vi "Write ADU Packet.vi"(8 "error in":errorcluster, 9 "modbus data unit":refnum<class "Modbus Data Unit.lvclass">, 10 "isMaster (f)":bool, 11 "ASCII transmission data unit in":refnum<class "ASCII Data Unit.lvclass">) -> (0 "error out":errorcluster, 3 "ASCII transmission data unit out":refnum<class "ASCII Data Unit.lvclass">)   [LabVIEW 2021, in "ASCII Data Unit.lvclass"]
uses:
  ASCII Data Unit.lvclass
  D:/my_projects/projects/Algorithms/Labview/21/Modbus_v121c/Transmission Data Unit/Serial Interface/Serial Data Unit.lvclass
  D:/my_projects/projects/Algorithms/Labview/21/Modbus_v121c/Transmission Data Unit/Transmission Data Unit.lvclass
  Modbus Data Unit/Modbus Data Unit.lvclass
  Modbus Data Unit/Modbus Data Unit.lvclass/Modbus Data Unit.ctl
  Serial Interface/Serial Data Unit.lvclass/Serial Data Unit.ctl
  Transmission Data Unit.lvclass/Transmission Data Unit.ctl
  <vilib>/Utility/error.llb/Error Cluster From Error Code.vi
  <vilib>/ErrorRing/Error Ring.xnode
  ASCII Data Unit.lvclass/ASCII Data Unit.ctl
  Serial Interface/Serial Data Unit.lvclass
  Transmission Data Unit.lvclass
  Network Interface/Serial Interface/Serial Shared Components/Serial Shared Components.lvlib
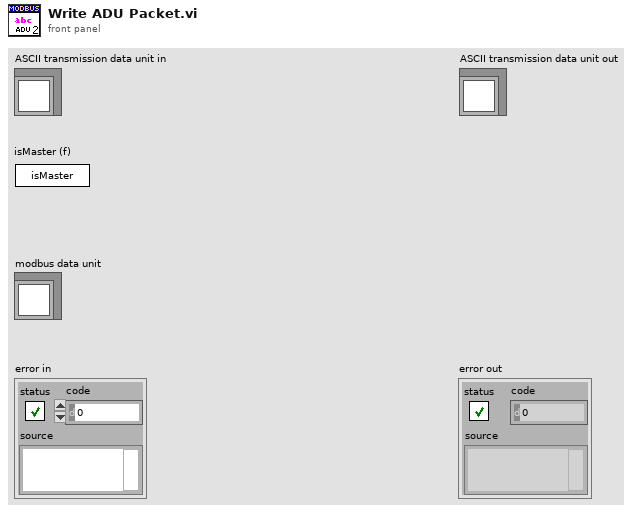
[diagram p1: front panel]
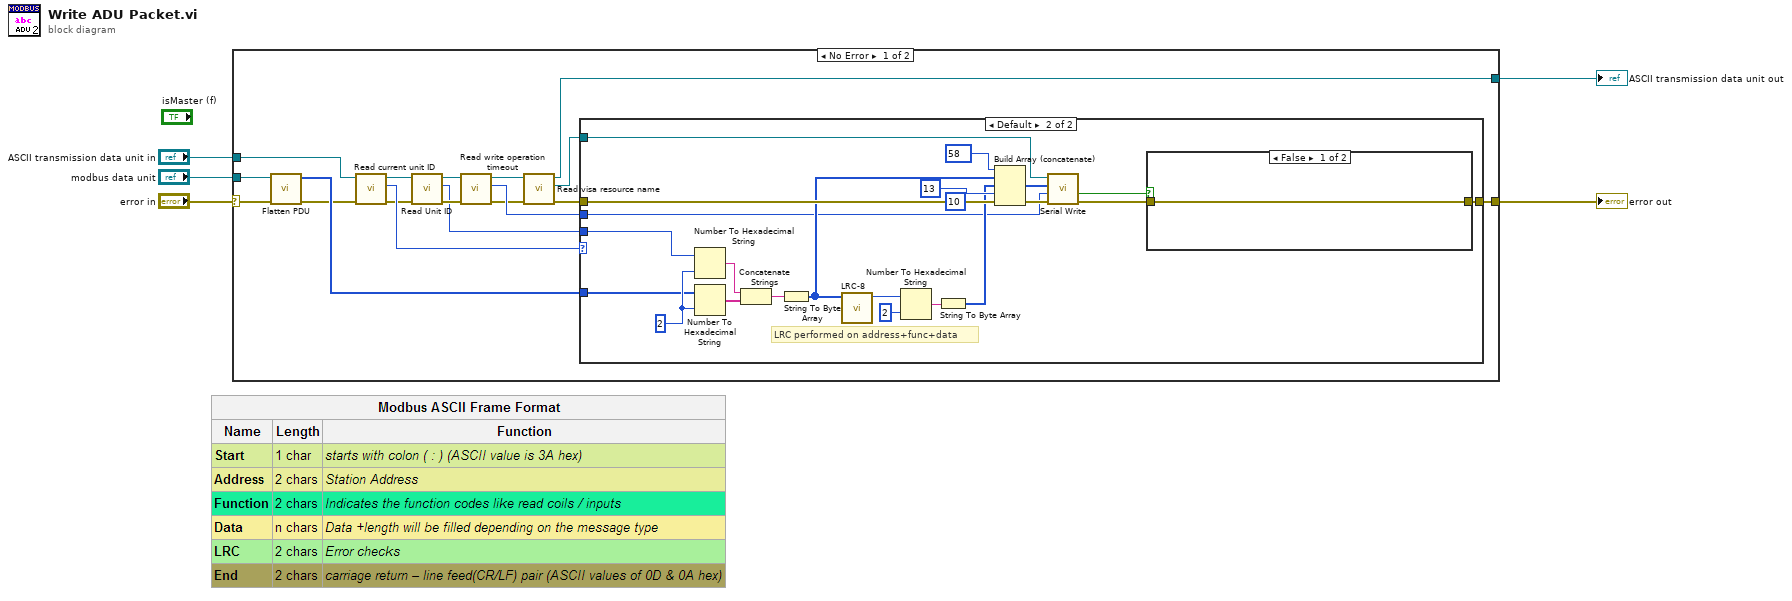
[diagram p0: block diagram]
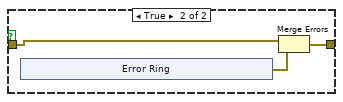
[diagram p3: hidden frame]
diagram:
  n1 = case shown="No Error" "error in" {
    selector: "error in" -> [w22 w55]
    tunnel: [w21 w55] -> w3
    tunnel: "modbus data unit" -> [w23 _]
    tunnel: "ASCII transmission data unit in" -> [w14 w54]
    tunnel: [w8 w54] -> w4
    frame No Error {
      n2 = call "Flatten PDU.vi"("error in"=w22, "modbus data unit in"=w23) -> ("error out"=w12:errorcluster, "Full modbus data unit"=w20:u8[])  [unwired: 8 in]
      n3 = call "Read current unit ID.vi"("error in (no error)"=w12, "Serial Data Unit in"=w14) -> ("error out"=w11:errorcluster, "request unit ID"=w15:u8, "Serial Data Unit out"=w13:refnum<class "ASCII Data Unit.lvclass">)  [unwired: 7 in]
      n4 = call "Read Unit ID.vi"("error in"=w11, "transmission data unit in"=w13) -> ("error out"=w19:errorcluster, "unit ID"=w16:u8, "transmission data unit out"=w18:refnum<class "ASCII Data Unit.lvclass">)  [unwired: 7 in]
      n5 = call "Read write operation timeout.vi"("error in (no error)"=w19, "transmission data unit in"=w18) -> ("error out"=w10:errorcluster, "write operation timeout"=w17:i32, "transmission data unit out"=w9:refnum<class "ASCII Data Unit.lvclass">)  [unwired: 7 in]
      n6 = call "Read visa resource name.vi"("error in (no error)"=w10, "Serial Data Unit in"=w9) -> ("error out"=w6:errorcluster, "visa resource name"=w7:refnum<visa-resource-name>, "Serial Data Unit out"=w8:refnum<class "ASCII Data Unit.lvclass">)  [unwired: 7 in]
      n7 = case shown="Default" w15 {
        tunnel: w7 -> [_ w45]
        tunnel: [w24 w42] -> w21
        tunnel: w16 -> [_ w40]
        tunnel: w20 -> [_ w39]
        tunnel: w6 -> [w24 w33]
        tunnel: w17 -> [_ w25]
        frame 0 {
          # "request unit ID defaults to 1. If it is 0 it was set that way. If it was set that way, this is a slave trying to respond to a broadcast"
        }
        frame Default {
          w41 = 2
          # "LRC performed on address+func+data"
          n8 = Number To Hexadecimal String(1:w41, 2:w40) -> (0:w37:string)
          n9 = Number To Hexadecimal String(1:w41, 2:w39) -> (0:w38:string[])
          n10 = Concatenate Strings(w37, w38) -> (w27:string)
          n11 = String To Byte Array(string=w27) -> (unsigned byte array=w26:u8[])
          n12 = call "LRC-8.vi"("data"=w26) -> ("LRC-8"=w35:u8)  [unwired: 10 in]
          n13 = Number To Hexadecimal String(1:i16 2 ("width (-)"), 2:w35) -> (0:w29:string)
          n14 = String To Byte Array(string=w29) -> (unsigned byte array=w28:u8[])
          n15 = Build Array (concatenate)(u8 58 ("element"), w26, w28, u8 13 ("element"), u8 10 ("element")) -> (w34:u8[])
          n16 = call "Serial Write.vi"("error in"=w33, "timeout (ms)"=w25, "data"=w34, "Visa Resource"=w45) -> ("error out"=w43:errorcluster, "timed out?"=w44:bool)  [unwired: 6 in]
          n17 = case shown="False" w44 {
            tunnel: w43 -> [w46 w48]
            tunnel: [w46 w49] -> w42
            frame False {
            }
            frame True {
              n18 = xnode "Error Ring"() -> ("error out"=w47:errorcluster)
              n19 = Merge Errors(w48, w47) -> (w49:errorcluster)
            }
          }
        }
      }
    }
    frame Error {
    }
  }
  "error out" <- w3
  "ASCII transmission data unit out" <- w4
